vi "Test Overflow.vi"(8 "error in":errorcluster, 11 "Test Case In":refnum<class "Undo Redo Core.lvclass">) -> (0 "error out":errorcluster, 3 "Test Case Out":refnum<class "Undo Redo Core.lvclass">)   [LabVIEW 2021, in "Undo Redo Core.lvclass"]
doc: "Adds many states to the undo buffer and then performs an Undo on all of the added states."
uses:
  Undo Redo Core.lvclass
  C:/Program Files/National Instruments/LabVIEW 2024/vi.lib/Astemes/LUnit/Test Case.lvclass
  <resource>/plugins/NIIconEditor/Controls/Undo Redo Action.ctl
  <vilib>/Astemes/LUnit/Test Case.lvclass/Test Case.ctl
  <vilib>/Astemes/LUnit/Append Fail Result.vi
  <vilib>/Astemes/LUnit/Append Pass Result.vi
  <vilib>/Astemes/LUnit/Run In UI.vi
  <vilib>/Utility/error.llb/Clear Errors.vi
  <vilib>/Astemes/LUnit/Test Case.lvclass
panel:
  out "Have Changes":bool
  out "Undo Data":string[](array[string])
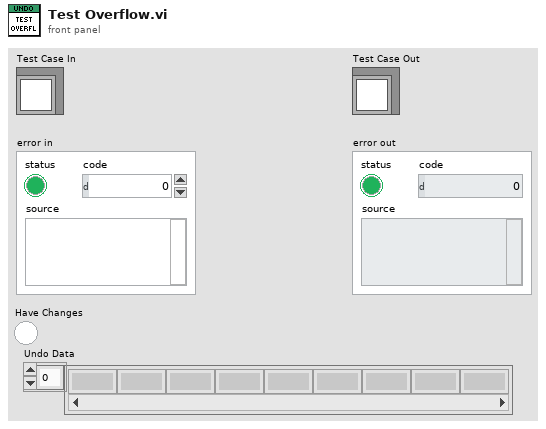
[diagram p1: front panel]
types:
  T1 = typedef "Undo Redo Action.ctl" = enum16{"Init", "Add", "Undo", "Redo", "Current State"}
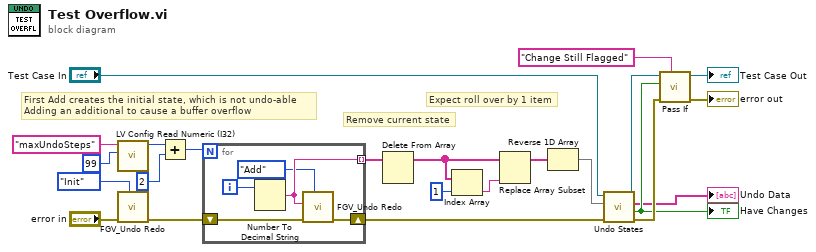
[diagram p0: block diagram]
diagram:
  # "Expect roll over by 1 item"
  # "Remove current state"
  # "First Add creates the initial state, which is not undo-able\nAdding an additional to cause a buffer overflow"
  n1 = call <resource>:"LV Config Read Numeric (I32).vi"("default value"=99, "key"="maxUndoSteps") -> ("value"=w14:i32)  [unwired: 3 in, 2 out]
  n2 = call <resource>:"FGV_Undo Redo.vi"("Action"=Undo_Redo_Action."Init", "error in"="error in") -> ("error out"=w20:errorcluster)  [unwired: 7 in, 2 out]
  n3 = Add(x=w14, y=2) -> (x+y=w13:i32)
  n4 = for {
    N: w13 -> [_]
    shift-right: [w27] -> w22
    shift-left: w20 -> [w28]
    tunnel: [w25] -> w10 mode=indexing
    i -> [w26]
    n5 = Number To Decimal String(number=w26) -> (decimal integer string=w25:string)  [unwired: 1 in]
    n6 = call <resource>:"FGV_Undo Redo.vi"("Action"=Undo_Redo_Action."Add", "error in"=w28, "State In"=w25) -> ("error out"=w27:errorcluster)  [unwired: 6 in, 2 out]
  }
  n7 = Delete From Array(array=w10) -> (array with subset deleted=w1:string[])  [unwired: 2 in, 1 out]
  n8 = Index Array(array=w1, index=1) -> (element=w8:string)
  n9 = Replace Array Subset(array=w1, new element=w8) -> (w7:string[])  [unwired: 1 in]
  n10 = Reverse 1D Array(array=w7) -> (reversed array=w2:string[])
  n11 = call "Undo States.vi"("error in"=w22, "Expected Undo States"=w2, "Test Case In"="Test Case In") -> ("error out"=w23:errorcluster, "Final Have Changes"=w18:bool, "Actual Undo States"=→"Undo Data":string[], "Test Case Out"=w5:refnum<class "Undo Redo Core.lvclass">)  [unwired: 5 in]
  "Have Changes" <- w18
  n12 = call <vilib>:"Pass If.vi"("Description"="Change Still Flagged", "error in (no error)"=w23, "Pass?"=w18, "LUnit Test Case In"=w5) -> ("error out"=→"error out":errorcluster, "LUnit Test Case Out"=→"Test Case Out":refnum<class "Undo Redo Core.lvclass">)  [unwired: 6 in]
